vi "Sub_CheckFrameIntegrity.vi"(1 "Received string":string) -> (0 "Is this valid frame?":bool)   [LabVIEW 2018]
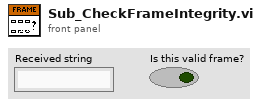
[diagram p1: front panel]
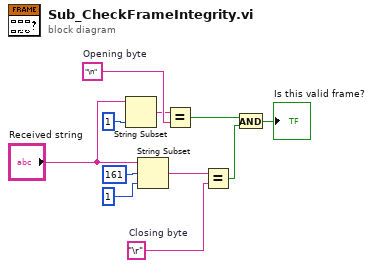
[diagram p0: block diagram]
diagram:
  w11 = "\r"  # Closing byte
  w6 = "\n"  # Opening byte
  n1 = String Subset(string="Received string", length (rest)=1 ("length (rest)")) -> (substring=w5:string)  [unwired: 1 in]
  n2 = String Subset(string="Received string", offset (0)=161, length (rest)=1 ("length (rest)")) -> (substring=w10:string)
  n3 = Equal?(x=w5, y=w6) -> (x = y?=w1:bool)
  n4 = Equal?(x=w10, y=w11) -> (x = y?=w2:bool)
  n5 = And(x=w1, y=w2) -> (x .and. y?=→"Is this valid frame?":bool)
